vi "Логи_UKF_probe.vi"() -> ()   [LabVIEW 2013]
panel:
  in  "Tab Control":T1(tab)
  out "pos":cluster{dbl[], dbl[]}[](graph)
  out "pos 2":cluster{dbl[], dbl[]}[](graph)
  out "vel":cluster{dbl[], dbl[]}[](graph)
  out "bias":cluster{dbl[], dbl[]}[](graph)
  out "angle":cluster{dbl[], dbl[]}[](graph)
  out "ID параметров":u8[](array[numeric])
  out "Длина заголовка":i32
  out "Заголовок":string
  out "Количество параметров":u8
  out "size (in bytes)":i64
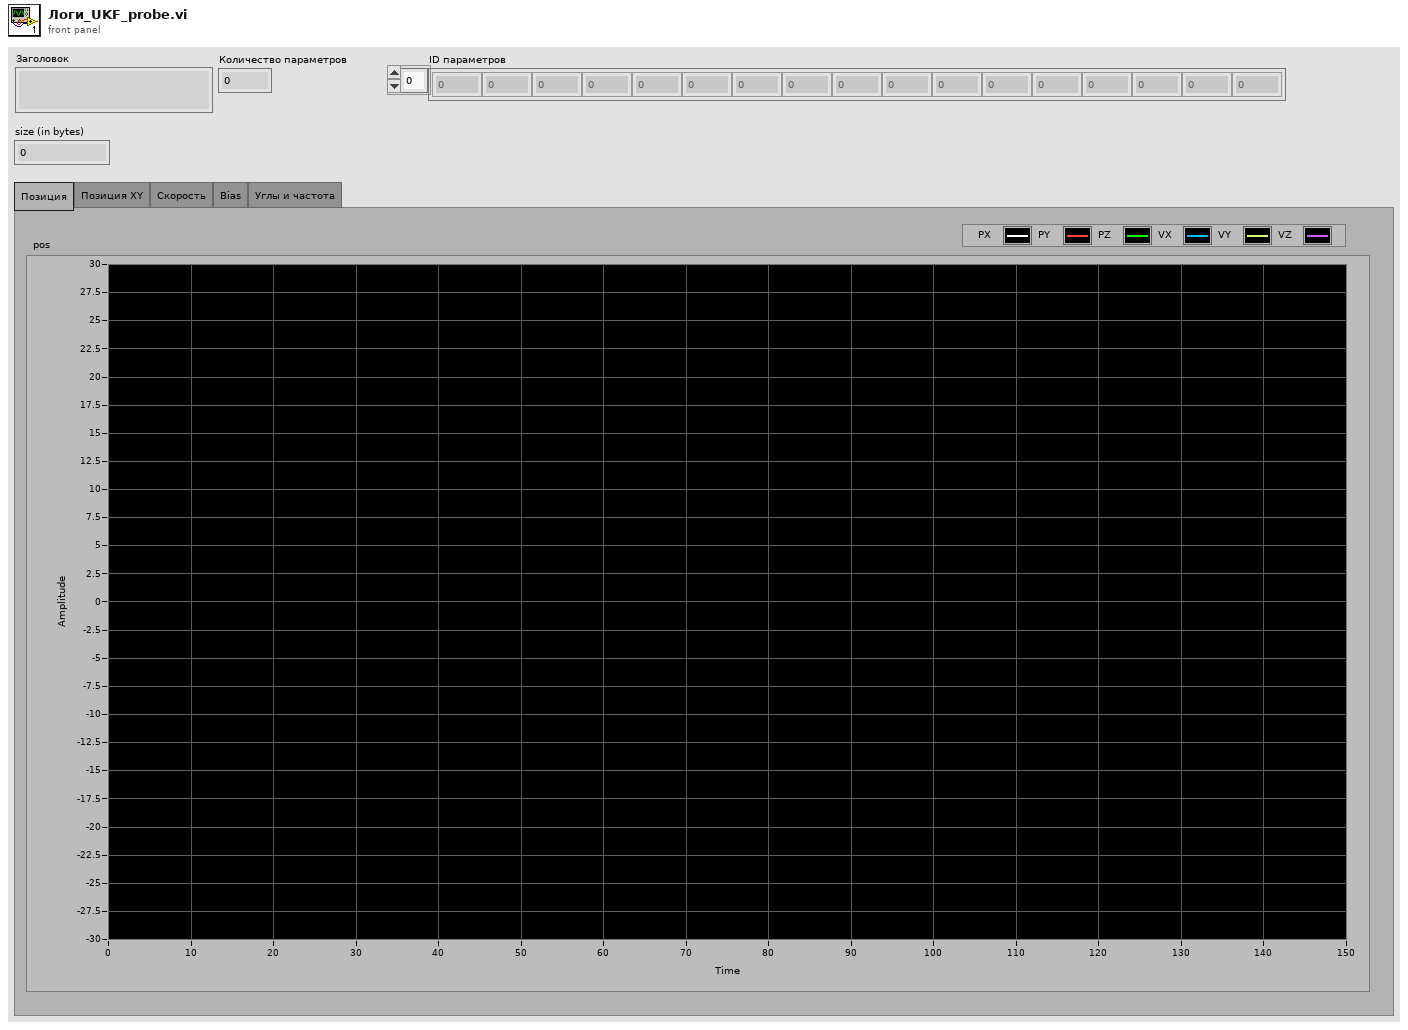
[diagram p1: front panel]
types:
  T1 = enum32{"Позиция", "Позиция XY", "Скорость", "Bias", "Углы и частота"}
  T2 = enum16{"open", "replace", "create", "open or create", "replace or create", "replace or create with confirmation"}
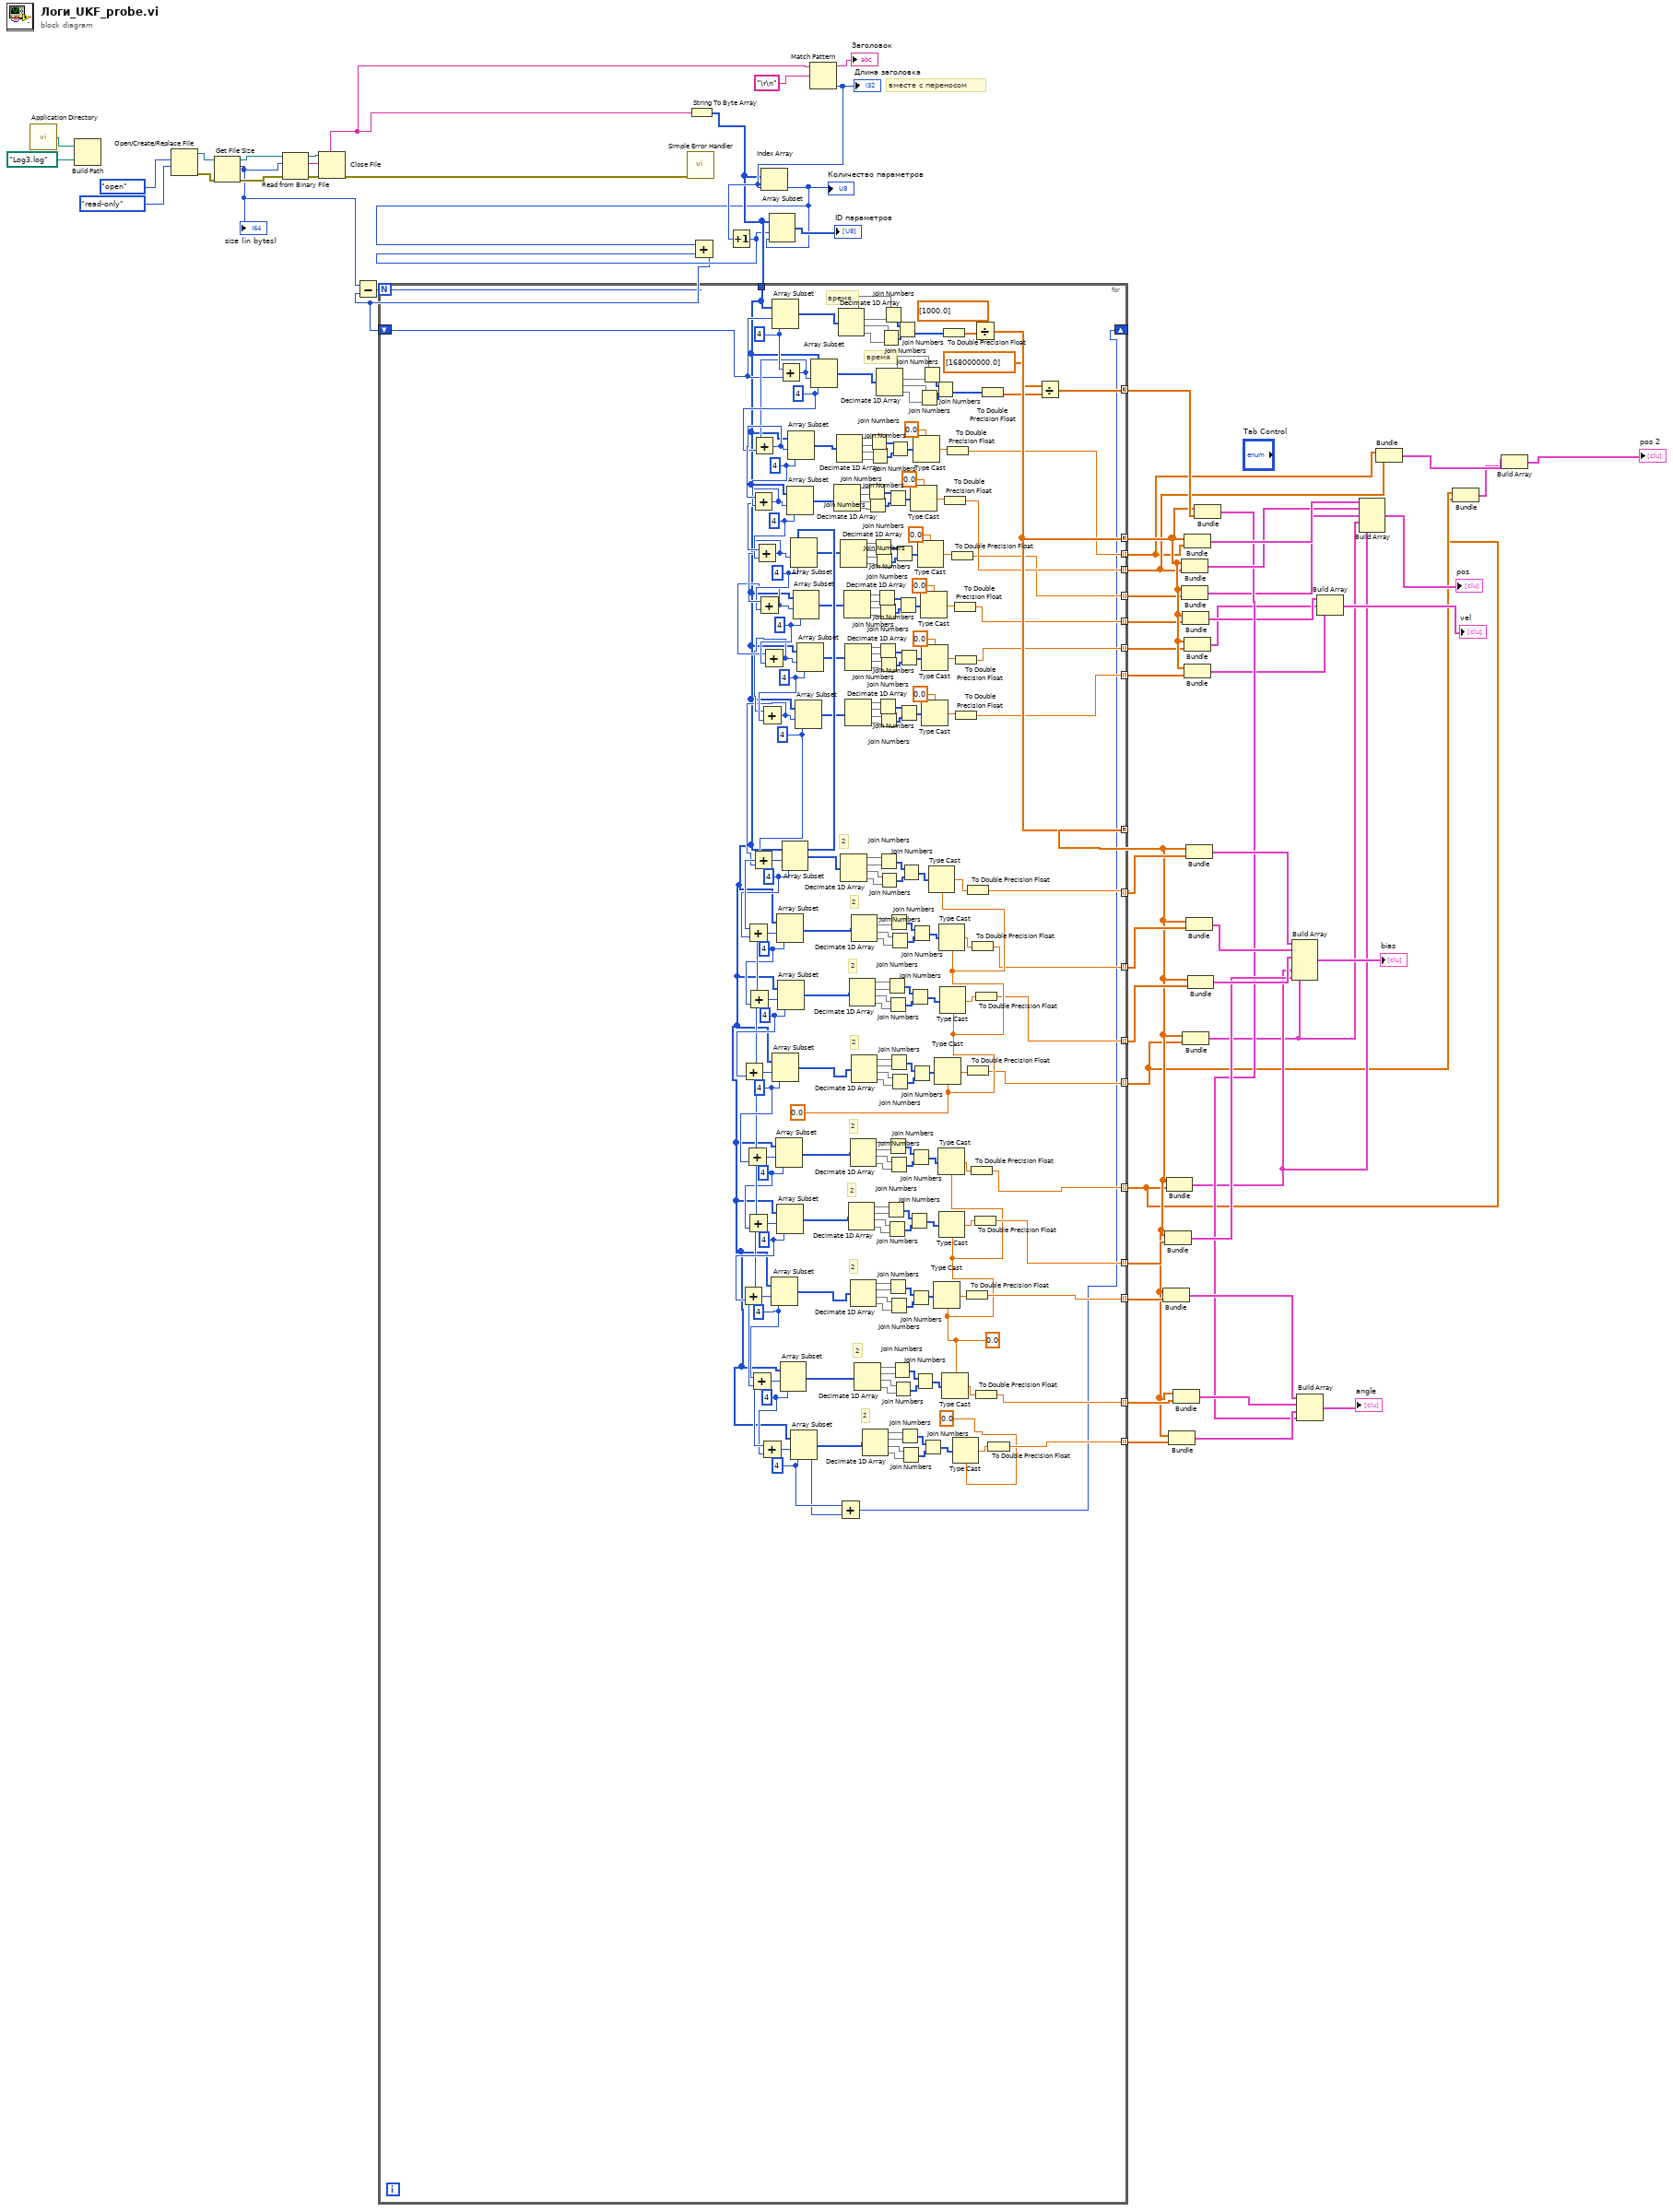
[diagram p0: block diagram]
diagram:
  # "вместе с переносом"
  n1 = call <vilib>:"Application Directory.vi"() -> ("Application Directory"=w60:path)
  n2 = Build Path(base path=w60, name or relative path=path "Log3.log" ("default name")) -> ()  [unwired: 1 out]
  n3 = Open/Create/Replace File(operation (0:open)=T2."open", access (0:read/write)=enum16{"read/write", "read-only", "write-only"}."read-only") -> (refnum out=w57:refnum<file>, error out=w55:errorcluster)  [unwired: 4 in, 1 out]
  n4 = Get File Size(file=w57, error in=w55) -> (refnum out=w56:refnum<file>, size (in bytes)=w47:i64, 0:w54:errorcluster)
  "size (in bytes)" <- w47
  n5 = Read from Binary File(8:w54, 10:w47, 11:w56) -> (0:w58:errorcluster, 2:w53:string, 3:w59:refnum<file>)  [unwired: 3 in, 1 out]
  n6 = Close File(refnum=w59, error in=w58) -> (error out=w63:errorcluster)  [unwired: 1 out]
  n7 = call <vilib>:"Simple Error Handler.vi"("error in (no error)"=w63) -> ()  [unwired: 4 in, 5 out]
  n8 = String To Byte Array(string=w53) -> (unsigned byte array=w48:u8[])
  n9 = Match Pattern(string=w53, regular expression="\r\n" ("format string")) -> (before substring=→"Заголовок":string, offset past match=w50:i32)  [unwired: 1 in, 2 out]
  "Длина заголовка" <- w50
  n10 = Increment(x=w50) -> (x+1=w45:i32)
  n11 = Index Array(array=w48, index=w50) -> (element=w46:u8)
  "Количество параметров" <- w46
  n12 = Add(x=w46, y=w45) -> (x+y=w44:i32)
  n13 = Subtract(x=w47, y=w44) -> (x-y=w43:i64)
  n14 = for {
    N: w43 -> [_]
    tunnel: w48 -> [w134]
    shift-right: [w64] -> _
    shift-left: w44 -> [w142]
    tunnel: [w221] -> w28 mode=concatenating
    tunnel: [w166] -> w31 mode=indexing
    tunnel: [w165] -> w32 mode=indexing
    tunnel: [w164] -> w33 mode=indexing
    tunnel: [w163] -> w3 mode=indexing
    tunnel: [w221] -> w37 mode=concatenating
    tunnel: [w183] -> w2 mode=indexing
    tunnel: [w182] -> w40 mode=indexing
    tunnel: [w181] -> w39 mode=indexing
    tunnel: [w167] -> w38 mode=concatenating
    tunnel: [w136] -> w30 mode=indexing
    tunnel: [w135] -> w29 mode=indexing
    tunnel: [w72] -> w6 mode=indexing
    tunnel: [w71] -> w10 mode=indexing
    tunnel: [w70] -> w27 mode=indexing
    tunnel: [w69] -> w26 mode=indexing
    tunnel: [w68] -> w25 mode=indexing
    tunnel: [w67] -> w24 mode=indexing
    w66 = 4 ("length")
    w161 = 4 ("length")
    w171 = 4 ("length")
    w139 = sgl 0.0
    w138 = 4 ("length")
    w216 = 4 ("length")
    w214 = 4 ("length")
    w141 = 4 ("length")
    w219 = 4 ("length")
    w220 = 4 ("length")
    w222 = 4 ("length")
    w224 = 4 ("length")
    w226 = 4 ("length")
    w230 = sgl 0.0
    w185 = 4 ("length")
    w278 = 4 ("length")
    w276 = 4 ("length")
    w279 = 4 ("length")
    w172 = 4 ("length")
    # "2"
    # "2"
    # "время"
    # "2"
    # "2"
    # "2"
    # "2"
    # "2"
    # "2"
    # "2"
    # "время"
    n15 = Array Subset(array=w134, index=w142, length=w172) -> (w265:u8[])
    n16 = Add(x=w172, y=w142) -> (x+y=w170:i32)
    n17 = Add(x=w170, y=w171) -> (x+y=w227:i32)
    n18 = Add(x=w227, y=w226) -> (x+y=w225:i32)
    n19 = Add(x=w225, y=w224) -> (x+y=w223:i32)
    n20 = Add(x=w223, y=w222) -> (x+y=w218:i32)
    n21 = Add(x=w218, y=w220) -> (x+y=w217:i32)
    n22 = Add(x=w217, y=w219) -> (x+y=w140:i32)
    n23 = Add(x=w141, y=w140) -> (x+y=w280:i32)
    n24 = Add(x=w280, y=w279) -> (x+y=w277:i32)
    n25 = Add(x=w277, y=w276) -> (x+y=w275:i32)
    n26 = Add(x=w275, y=w278) -> (x+y=w184:i32)
    n27 = Add(x=w184, y=w185) -> (x+y=w215:i32)
    n28 = Add(x=w215, y=w214) -> (x+y=w213:i32)
    n29 = Add(x=w213, y=w216) -> (x+y=w137:i32)
    n30 = Add(x=w138, y=w137) -> (x+y=w162:i32)
    n31 = Add(x=w162, y=w161) -> (x+y=w65:i32)
    n32 = Array Subset(array=w134, index=w137, length=w138) -> (w192:u8[])
    n33 = Array Subset(array=w134, index=w184, length=w185) -> (w238:u8[])
    n34 = Array Subset(array=w134, index=w215, length=w214) -> (w206:u8[])
    n35 = Array Subset(array=w134, index=w277, length=w276) -> (w252:u8[])
    n36 = Array Subset(array=w134, index=w213, length=w216) -> (w199:u8[])
    n37 = Array Subset(array=w134, index=w275, length=w278) -> (w245:u8[])
    n38 = Array Subset(array=w134, index=w162, length=w161) -> (w154:u8[])
    n39 = Array Subset(array=w134, index=w280, length=w279) -> (w266:u8[])
    n40 = Array Subset(array=w134, index=w225, length=w224) -> (w77:u8[])
    n41 = Array Subset(array=w134, index=w227, length=w226) -> (w124:u8[])
    n42 = Array Subset(array=w134, index=w223, length=w222) -> (w76:u8[])
    n43 = Array Subset(array=w134, index=w65, length=w66) -> (w147:u8[])
    n44 = Array Subset(array=w134, index=w218, length=w220) -> (w75:u8[])
    n45 = Array Subset(array=w134, index=w140, length=w141) -> (w73:u8[])
    n46 = Array Subset(array=w134, index=w217, length=w219) -> (w74:u8[])
    n47 = Array Subset(array=w134, index=w170, length=w171) -> (w174:u8[])
    n48 = Decimate 1D Array(w77) -> (w121:u8[], w122:u8[], w120:u8[], w119:u8[])
    n49 = Decimate 1D Array(w124) -> (w131:u8[], w132:u8[], w130:u8[], w129:u8[])
    n50 = Add(x=w66, y=w65) -> (x+y=w64:i32)
    n51 = Decimate 1D Array(w265) -> (w268:u8[], w269:u8[], w270:u8[], w271:u8[])
    n52 = Decimate 1D Array(w76) -> (w112:u8[], w113:u8[], w111:u8[], w110:u8[])
    n53 = Decimate 1D Array(w266) -> (w273:u8[], w274:u8[], w262:u8[], w261:u8[])
    n54 = Decimate 1D Array(w75) -> (w103:u8[], w104:u8[], w102:u8[], w101:u8[])
    n55 = Decimate 1D Array(w74) -> (w94:u8[], w95:u8[], w93:u8[], w92:u8[])
    n56 = Decimate 1D Array(w73) -> (w85:u8[], w86:u8[], w84:u8[], w83:u8[])
    n57 = Decimate 1D Array(w199) -> (w204:u8[], w205:u8[], w203:u8[], w202:u8[])
    n58 = Decimate 1D Array(w245) -> (w250:u8[], w251:u8[], w249:u8[], w248:u8[])
    n59 = Decimate 1D Array(w206) -> (w211:u8[], w212:u8[], w210:u8[], w209:u8[])
    n60 = Decimate 1D Array(w192) -> (w197:u8[], w198:u8[], w196:u8[], w195:u8[])
    n61 = Decimate 1D Array(w252) -> (w257:u8[], w258:u8[], w256:u8[], w255:u8[])
    n62 = Decimate 1D Array(w238) -> (w243:u8[], w244:u8[], w242:u8[], w241:u8[])
    n63 = Decimate 1D Array(w154) -> (w159:u8[], w160:u8[], w158:u8[], w157:u8[])
    n64 = Decimate 1D Array(w147) -> (w152:u8[], w153:u8[], w151:u8[], w150:u8[])
    n65 = Join Numbers(hi=w121, lo=w122) -> ((hi.lo)=w118:u16[])
    n66 = Join Numbers(hi=w120, lo=w119) -> ((hi.lo)=w117:u16[])
    n67 = Join Numbers(hi=w131, lo=w132) -> ((hi.lo)=w128:u16[])
    n68 = Join Numbers(hi=w130, lo=w129) -> ((hi.lo)=w127:u16[])
    n69 = Join Numbers(hi=w112, lo=w113) -> ((hi.lo)=w109:u16[])
    n70 = Join Numbers(hi=w111, lo=w110) -> ((hi.lo)=w108:u16[])
    n71 = Join Numbers(hi=w103, lo=w104) -> ((hi.lo)=w100:u16[])
    n72 = Join Numbers(hi=w102, lo=w101) -> ((hi.lo)=w99:u16[])
    n73 = Join Numbers(hi=w94, lo=w95) -> ((hi.lo)=w91:u16[])
    n74 = Join Numbers(hi=w85, lo=w86) -> ((hi.lo)=w82:u16[])
    n75 = Join Numbers(hi=w93, lo=w92) -> ((hi.lo)=w90:u16[])
    n76 = Join Numbers(hi=w84, lo=w83) -> ((hi.lo)=w81:u16[])
    n77 = Join Numbers(hi=w273, lo=w274) -> ((hi.lo)=w260:u16[])
    n78 = Decimate 1D Array(w174) -> (w176:u8[], w177:u8[], w178:u8[], w179:u8[])
    n79 = Join Numbers(hi=w262, lo=w261) -> ((hi.lo)=w259:u16[])
    n80 = Join Numbers(hi=w270, lo=w271) -> ((hi.lo)=w267:u16[])
    n81 = Join Numbers(hi=w268, lo=w269) -> ((hi.lo)=w272:u16[])
    n82 = Join Numbers(hi=w204, lo=w205) -> ((hi.lo)=w201:u16[])
    n83 = Join Numbers(hi=w250, lo=w251) -> ((hi.lo)=w247:u16[])
    n84 = Join Numbers(hi=w203, lo=w202) -> ((hi.lo)=w200:u16[])
    n85 = Join Numbers(hi=w118, lo=w117) -> ((hi.lo)=w116:u32[])
    n86 = Join Numbers(hi=w249, lo=w248) -> ((hi.lo)=w246:u16[])
    n87 = Join Numbers(hi=w211, lo=w212) -> ((hi.lo)=w208:u16[])
    n88 = Join Numbers(hi=w197, lo=w198) -> ((hi.lo)=w194:u16[])
    n89 = Join Numbers(hi=w257, lo=w258) -> ((hi.lo)=w254:u16[])
    n90 = Join Numbers(hi=w243, lo=w244) -> ((hi.lo)=w240:u16[])
    n91 = Join Numbers(hi=w210, lo=w209) -> ((hi.lo)=w207:u16[])
    n92 = Join Numbers(hi=w196, lo=w195) -> ((hi.lo)=w193:u16[])
    n93 = Join Numbers(hi=w256, lo=w255) -> ((hi.lo)=w253:u16[])
    n94 = Join Numbers(hi=w242, lo=w241) -> ((hi.lo)=w239:u16[])
    n95 = Join Numbers(hi=w128, lo=w127) -> ((hi.lo)=w126:u32[])
    n96 = Join Numbers(hi=w159, lo=w160) -> ((hi.lo)=w156:u16[])
    n97 = Join Numbers(hi=w158, lo=w157) -> ((hi.lo)=w155:u16[])
    n98 = Join Numbers(hi=w109, lo=w108) -> ((hi.lo)=w107:u32[])
    n99 = Join Numbers(hi=w272, lo=w267) -> ((hi.lo)=w233:u32[])
    n100 = Join Numbers(hi=w100, lo=w99) -> ((hi.lo)=w98:u32[])
    n101 = Join Numbers(hi=w91, lo=w90) -> ((hi.lo)=w89:u32[])
    n102 = Join Numbers(hi=w82, lo=w81) -> ((hi.lo)=w80:u32[])
    n103 = Join Numbers(hi=w152, lo=w153) -> ((hi.lo)=w149:u16[])
    n104 = Join Numbers(hi=w151, lo=w150) -> ((hi.lo)=w148:u16[])
    n105 = Join Numbers(hi=w260, lo=w259) -> ((hi.lo)=w229:u32[])
    n106 = Join Numbers(hi=w201, lo=w200) -> ((hi.lo)=w189:u32[])
    n107 = Join Numbers(hi=w247, lo=w246) -> ((hi.lo)=w235:u32[])
    n108 = Join Numbers(hi=w208, lo=w207) -> ((hi.lo)=w187:u32[])
    n109 = Join Numbers(hi=w194, lo=w193) -> ((hi.lo)=w190:u32[])
    n110 = Join Numbers(hi=w254, lo=w253) -> ((hi.lo)=w232:u32[])
    n111 = Join Numbers(hi=w240, lo=w239) -> ((hi.lo)=w236:u32[])
    n112 = Type Cast(type=sgl 0.0, x=w116) -> (*(type *) &x=w115:sgl)
    n113 = Join Numbers(hi=w156, lo=w155) -> ((hi.lo)=w144:u32[])
    n114 = Type Cast(type=sgl 0.0, x=w126) -> (*(type *) &x=w125:sgl)
    n115 = Join Numbers(hi=w178, lo=w179) -> ((hi.lo)=w175:u16[])
    n116 = Type Cast(type=sgl 0.0, x=w107) -> (*(type *) &x=w106:sgl)
    n117 = Join Numbers(hi=w176, lo=w177) -> ((hi.lo)=w180:u16[])
    n118 = Join Numbers(hi=w149, lo=w148) -> ((hi.lo)=w146:u32[])
    n119 = Type Cast(type=sgl 0.0, x=w98) -> (*(type *) &x=w97:sgl)
    n120 = Type Cast(type=sgl 0.0, x=w89) -> (*(type *) &x=w88:sgl)
    n121 = Type Cast(type=sgl 0.0, x=w80) -> (*(type *) &x=w79:sgl)
    n122 = Type Cast(type=w230, x=w229) -> (*(type *) &x=w228:sgl)
    n123 = Join Numbers(hi=w180, lo=w175) -> ((hi.lo)=w173:u32[])
    n124 = Type Cast(type=w139, x=w190) -> (*(type *) &x=w191:sgl)
    n125 = Type Cast(type=w230, x=w236) -> (*(type *) &x=w237:sgl)
    n126 = Type Cast(type=w139, x=w187) -> (*(type *) &x=w186:sgl)
    n127 = Type Cast(type=w230, x=w232) -> (*(type *) &x=w231:sgl)
    n128 = Type Cast(type=w139, x=w189) -> (*(type *) &x=w188:sgl)
    n129 = Type Cast(type=w230, x=w235) -> (*(type *) &x=w234:sgl)
    n130 = To Double Precision Float(number=w233) -> (double precision float=w264:dbl[])
    n131 = To Double Precision Float(number=w115) -> (double precision float=w71:dbl)
    n132 = Type Cast(type=w139, x=w144) -> (*(type *) &x=w143:sgl)
    n133 = To Double Precision Float(number=w125) -> (double precision float=w72:dbl)
    n134 = To Double Precision Float(number=w106) -> (double precision float=w70:dbl)
    n135 = To Double Precision Float(number=w97) -> (double precision float=w69:dbl)
    n136 = Type Cast(type=sgl 0.0, x=w146) -> (*(type *) &x=w145:sgl)
    n137 = To Double Precision Float(number=w88) -> (double precision float=w68:dbl)
    n138 = To Double Precision Float(number=w79) -> (double precision float=w67:dbl)
    n139 = To Double Precision Float(number=w191) -> (double precision float=w181:dbl)
    n140 = To Double Precision Float(number=w228) -> (double precision float=w166:dbl)
    n141 = To Double Precision Float(number=w237) -> (double precision float=w163:dbl)
    n142 = To Double Precision Float(number=w186) -> (double precision float=w183:dbl)
    n143 = To Double Precision Float(number=w231) -> (double precision float=w165:dbl)
    n144 = Divide(x=w264, y=dbl[] [1000.0]) -> (x/y=w221:dbl[])
    n145 = To Double Precision Float(number=w188) -> (double precision float=w182:dbl)
    n146 = To Double Precision Float(number=w234) -> (double precision float=w164:dbl)
    n147 = To Double Precision Float(number=w143) -> (double precision float=w136:dbl)
    n148 = To Double Precision Float(number=w173) -> (double precision float=w169:dbl[])
    n149 = To Double Precision Float(number=w145) -> (double precision float=w135:dbl)
    n150 = Divide(x=dbl[] [168000000.0] ("y"), y=w169) -> (x/y=w167:dbl[])
  }
  n151 = Array Subset(array=w48, index=w45, length=w46) -> (→"ID параметров":u8[])
  n152 = Bundle(w28, w39) -> (w17:cluster{dbl[], dbl[]})  [unwired: 1 in]
  n153 = Bundle(w28, w40) -> (w20:cluster{dbl[], dbl[]})  [unwired: 1 in]
  n154 = Bundle(w28, w2) -> (w7:cluster{dbl[], dbl[]})  [unwired: 1 in]
  n155 = Bundle(w28, w29) -> (w15:cluster{dbl[], dbl[]})  [unwired: 1 in]
  n156 = Bundle(w28, w30) -> (w16:cluster{dbl[], dbl[]})  [unwired: 1 in]
  n157 = Bundle(w37, w10) -> (w22:cluster{dbl[], dbl[]})  [unwired: 1 in]
  n158 = Bundle(w37, w27) -> (w5:cluster{dbl[], dbl[]})  [unwired: 1 in]
  n159 = Bundle(w37, w26) -> (w13:cluster{dbl[], dbl[]})  [unwired: 1 in]
  n160 = Bundle(w28, w3) -> (w4:cluster{dbl[], dbl[]})  [unwired: 1 in]
  n161 = Bundle(w37, w6) -> (w23:cluster{dbl[], dbl[]})  [unwired: 1 in]
  n162 = Bundle(w37, w25) -> (w12:cluster{dbl[], dbl[]})  [unwired: 1 in]
  n163 = Bundle(w37, w24) -> (w11:cluster{dbl[], dbl[]})  [unwired: 1 in]
  n164 = Bundle(w28, w31) -> (w36:cluster{dbl[], dbl[]})  [unwired: 1 in]
  n165 = Bundle(w28, w32) -> (w35:cluster{dbl[], dbl[]})  [unwired: 1 in]
  n166 = Bundle(w28, w33) -> (w34:cluster{dbl[], dbl[]})  [unwired: 1 in]
  n167 = Bundle(w37, w38) -> (w14:cluster{dbl[], dbl[]})  [unwired: 1 in]
  n168 = Build Array(w36, w35, w34, w4, w7, w20) -> (→"bias":cluster{dbl[], dbl[]}[])
  n169 = Build Array(w17, w16, w15, w14) -> (→"angle":cluster{dbl[], dbl[]}[])
  n170 = Build Array(w13, w12, w11) -> (→"vel":cluster{dbl[], dbl[]}[])
  n171 = Build Array(w23, w22, w5, w4, w7) -> (→"pos":cluster{dbl[], dbl[]}[])
  n172 = Bundle(w6, w10) -> (w9:cluster{dbl[], dbl[]})  [unwired: 1 in]
  n173 = Bundle(w3, w2) -> (w1:cluster{dbl[], dbl[]})  [unwired: 1 in]
  n174 = Build Array(w9, w1) -> (→"pos 2":cluster{dbl[], dbl[]}[])
